vi "Data Source.vi"() -> (0 "Elements":i16[](array[numeric]))   [LabVIEW 2013]
doc: "This VI is a placeholder. Replace this VI or it's contents with your own code."
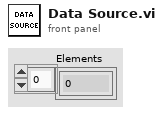
[diagram p1: front panel]
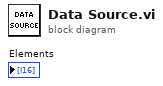
[diagram p0: block diagram]
diagram:
